vi "_TangoDeviceAttributesInfo.vi"(2 "error in":errorcluster, 3 "device name":string) -> (0 "error out":errorcluster, 1 "attributes_info":T1[](array[typedef]))   [LabVIEW 2014, in "tango.lvlib"]
uses:
  tango.lvlib
  Common VIs/Typedefs/_AttributeInfo_t.ctl
  Common VIs/Typedefs/_AttributeAccess_t.ctl
  Common VIs/Typedefs/_AttributeFormat_t.ctl
  Common VIs/Typedefs/_TangoDataType_t.ctl
  Common VIs/Typedefs/_AttributeLevel_t.ctl
  tango_binding.so
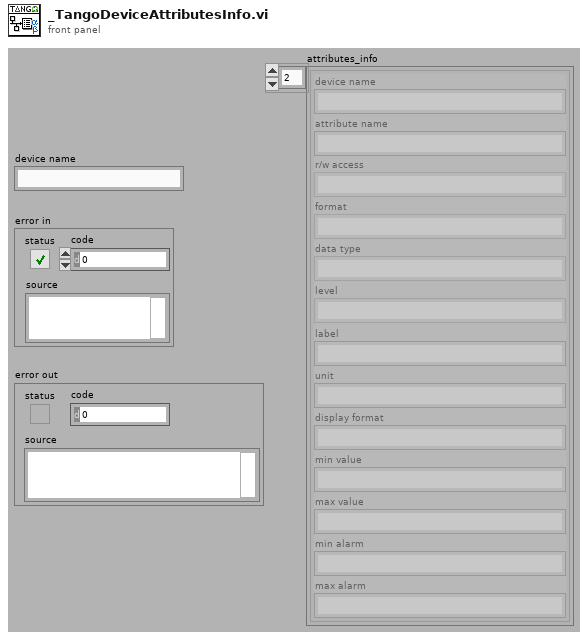
[diagram p1: front panel]
types:
  T1 = typedef "tango.lvlib/_AttributeInfo_t.ctl" = cluster{"device name":string, "attribute name":string, "r/w access":T2, "format":T3, "data type":T4, "level":T5, "label":string, "unit":string, "display format":string, "min value":string, "max value":string, "min alarm":string, "max alarm":string}
  T2 = typedef "tango.lvlib/_AttributeAccess_t.ctl" = enum16{"READ", "READ_WITH_WRITE", "WRITE", "READ_WRITE", "UNKNOWN_ACCESS_TYPE"}
  T3 = typedef "tango.lvlib/_AttributeFormat_t.ctl" = enum16{"SCALAR", "SPECTRUM", "IMAGE", "UNKNOWN_FORMAT"}
  T4 = typedef "tango.lvlib/_TangoDataType_t.ctl" = enum16{"VOID", "BOOLEAN", "SHORT", "LONG", "FLOAT", "DOUBLE", "USHORT", "ULONG", "STRING", "CHAR_ARRAY", "SHORT_ARRAY", "LONG_ARRAY", "FLOAT_ARRAY", "DOUBLE_ARRAY", "USHORT_ARRAY", "ULONG_ARRAY", "STRING_ARRAY", "LONG_STRING_ARRAY", "DOUBLE_STRING_ARRAY", "STATE", "CONST_STRING", "BOOLEAN_ARRAY", "UCHAR", "LONG64", "ULONG64", "LONG64_ARRAY", "ULONG64_ARRAY", "INT (not supported)", "ENCODED (not supported)", "ENUM", "PIPE_BLOB (not supported)", "STATE_ARRAY", "UNKNOW_DATA_TYPE"}
  T5 = typedef "tango.lvlib/_AttributeLevel_t.ctl" = enum16{"OPERATOR", "EXPERT", "UNKNOWN_LEVEL"}
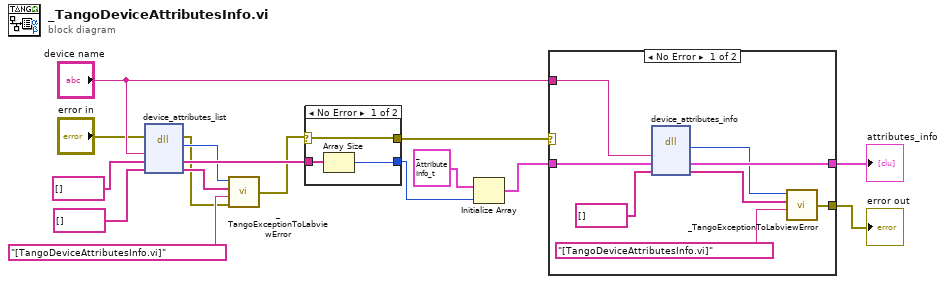
[diagram p0: block diagram]
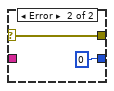
[diagram p3: hidden frame]
diagram:
  n1 = dll-call lib="tango_binding.*" fn="device_attributes_list"(error in="error in", "dev_name"="device name", "attributes_list"=string[] [] ("Error Stack"), "error_stack"=string[] [] ("Error Stack")) -> (error out=w4:errorcluster, "return type"=w7:i32, "attributes_list"=w16:string[], "error_stack"=w6:string[])  [unwired: 3 in, 1 out]
  n2 = call "_TangoExceptionToLabviewError.vi"("error in"=w4, "location"="[TangoDeviceAttributesInfo.vi]", "error stack"=w6, "error code"=w7) -> ("error out"=w13:errorcluster)
  n3 = case shown="No Error" w13 {
    selector: w13 -> [w18 w21]
    tunnel: w16 -> [w19 _]
    tunnel: [w18 w21] -> w12
    tunnel: [w17 0] -> w2
    frame No Error {
      n4 = Array Size(array=w19) -> (size(s)=w17:i32)
    }
    frame Error {
    }
  }
  n5 = Initialize Array(T1 {"device name"="", "attribute name"="", "r/w access"=enum."READ", "format"=enum."SCALAR", "data type"=enum."VOID", "level"=enum."OPERATOR", "label"="", "unit"="", "display format"="", "min value"="", "max value"="", "min alarm"="", "max alarm"=""} ("attribute info"), w2) -> (w1:T1[])
  n6 = case shown="No Error" w12 {
    selector: w12 -> [_ w31]
    tunnel: w1 -> [w28 w30]
    tunnel: [w27 w30] -> w10
    tunnel: "device name" -> [w22 _]
    tunnel: [w23 w31] -> w11
    frame No Error {
      n7 = dll-call lib="tango_binding.*" fn="device_attributes_info"("dev_name"=w22, "attributes_info"=w28, "error_stack"=string[] [] ("Error Stack")) -> ("return type"=w24:i32, "attributes_info"=w27:T1[], "error_stack"=w25:string[])  [unwired: 4 in, 2 out]
      n8 = call "_TangoExceptionToLabviewError.vi"("location"="[TangoDeviceAttributesInfo.vi]", "error stack"=w25, "error code"=w24) -> ("error out"=w23:errorcluster)  [unwired: 1 in]
    }
    frame Error {
    }
  }
  "error out" <- w11
  "attributes_info" <- w10
